vi "Get Name.vi"(8 "error in (no error)":errorcluster {"code" format="Error %.0f"}, 11 "GUI Documentation In":refnum<class "GUI Documentation.lvclass">) -> (0 "error out":errorcluster {"code" format="Error %.0f"}, 2 "Name":string, 3 "GUI Documentation Out":refnum<class "GUI Documentation.lvclass">)   [LabVIEW 2023, in "VIDoc Parsing.lvlib" / "GUI Documentation.lvclass"]
uses:
  GUI Documentation.lvclass
  GUI Documentation.lvclass/GUI Documentation.ctl
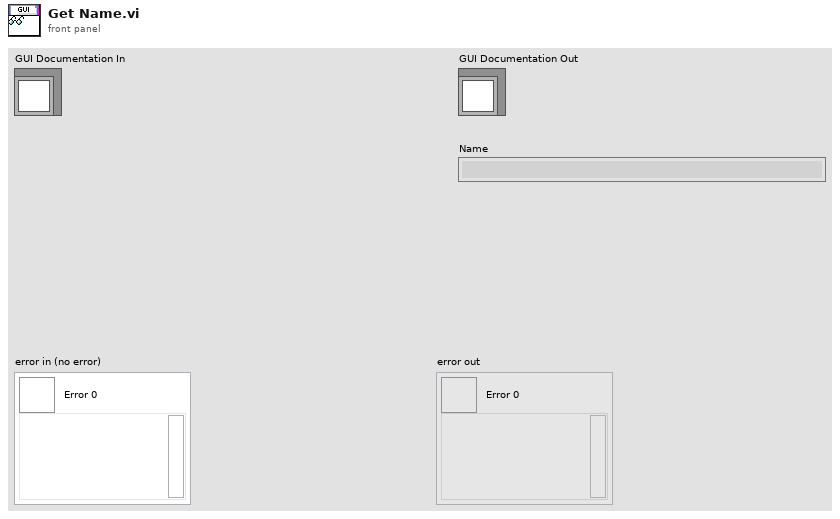
[diagram p1: front panel]
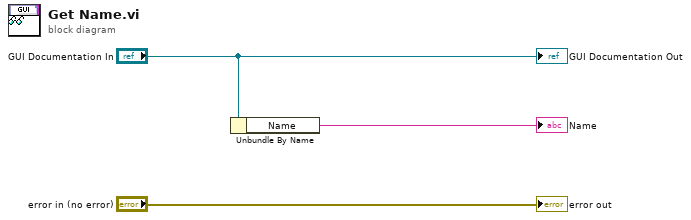
[diagram p0: block diagram]
diagram:
  n1 = Unbundle By Name("GUI Documentation In") -> ("Name"=→"Name":string)
  "error out" <- "error in (no error)"
  "GUI Documentation Out" <- "GUI Documentation In"
